vi "Test Each Driver.vi"() -> ()   [LabVIEW 2019, in "instrument.Cryostation.lvclass"]
uses:
  instrument.Cryostation.lvclass
panel:
  out "DBL":dbl
  in  "Enum":T1(ring)
  in  "address":string="130.49.180.32"
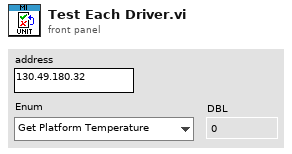
[diagram p1: front panel]
types:
  T1 = enum16{"Get Platform Temperature", "Get Sample Temperature", "Get Stage 1 Temperature", "Get Stage 2 Temperature", "Get Chamber Pressure"}
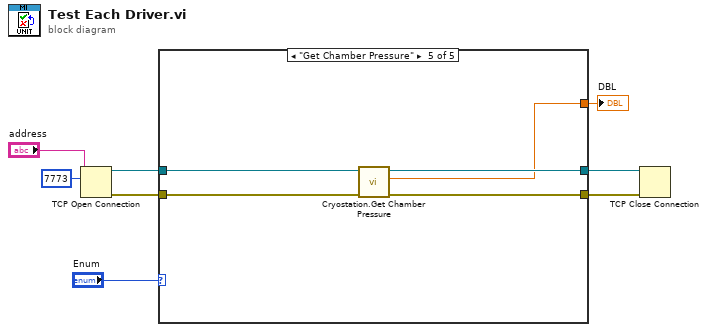
[diagram p0: block diagram]
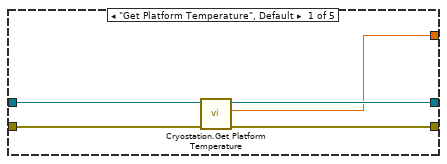
[diagram p2: hidden frame]
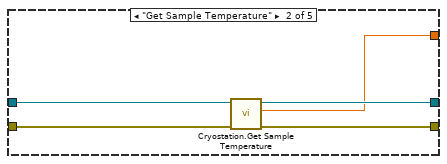
[diagram p3: hidden frame]
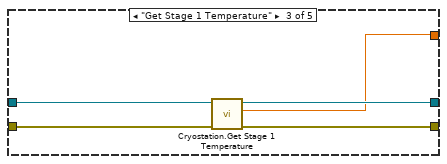
[diagram p4: hidden frame]
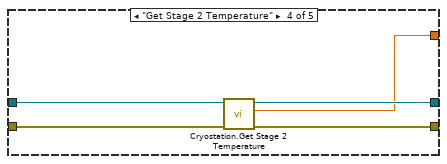
[diagram p5: hidden frame]
diagram:
  n1 = TCP Open Connection(address="address", remote port or service name=u16 7773) -> (connection ID=w3:refnum<k5>, error out=w5:errorcluster)  [unwired: 3 in]
  n2 = case shown="\"Get Chamber Pressure\"" "Enum" {
    tunnel: w5 -> [w13 w18 w23 w28 w33]
    tunnel: [w12 w16 w21 w26 w31] -> w4
    tunnel: w3 -> [w11 w17 w22 w27 w32]
    tunnel: [w10 w15 w20 w25 w30] -> w2
    tunnel: [w9 w14 w19 w24 w29] -> w1
    frame "Get Platform Temperature", Default {
      n3 = call "Cryostation.Get Platform Temperature.vi"("error in (no error)"=w13, "TCP Network Connection in"=w11) -> ("error out"=w12:errorcluster, "Platform Temperature (K)"=w9:dbl, "TCP Network Connection out"=w10:refnum<k5>)  [unwired: 7 in]
    }
    frame "Get Sample Temperature" {
      n4 = call "Cryostation.Get Sample Temperature.vi"("error in (no error)"=w18, "TCP Network Connection in"=w17) -> ("error out"=w16:errorcluster, "Sample Temperature (K)"=w14:dbl, "TCP Network Connection out"=w15:refnum<k5>)  [unwired: 7 in]
    }
    frame "Get Stage 1 Temperature" {
      n5 = call "Cryostation.Get Stage 1 Temperature.vi"("error in (no error)"=w23, "TCP Network Connection in"=w22) -> ("error out"=w21:errorcluster, "Stage 1 Temperature (K)"=w19:dbl, "TCP Network Connection out"=w20:refnum<k5>)  [unwired: 7 in]
    }
    frame "Get Stage 2 Temperature" {
      n6 = call "Cryostation.Get Stage 2 Temperature.vi"("error in (no error)"=w28, "TCP Network Connection in"=w27) -> ("error out"=w26:errorcluster, "Stage 2 Temperature (K)"=w24:dbl, "TCP Network Connection out"=w25:refnum<k5>)  [unwired: 7 in]
    }
    frame "Get Chamber Pressure" {
      n7 = call "Cryostation.Get Chamber Pressure.vi"("error in (no error)"=w33, "TCP Network Connection in"=w32) -> ("error out"=w31:errorcluster, "Chamber Pressure (mTorr)"=w29:dbl, "TCP Network Connection out"=w30:refnum<k5>)  [unwired: 7 in]
    }
  }
  "DBL" <- w1
  n8 = TCP Close Connection(connection ID=w2, error in (no error)=w4) -> ()  [unwired: 1 in, 2 out]
